vi "Lower First Letter.vi"(10 "String In":string) -> (2 "String Out":string)   [LabVIEW 2015, in "Case Manipulation.lvlib"]
uses:
  Case Manipulation.lvlib
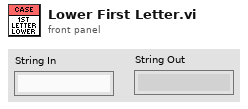
[diagram p1: front panel]
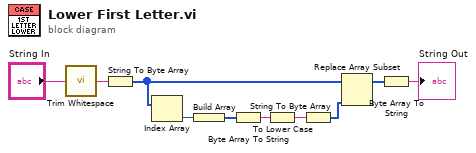
[diagram p0: block diagram]
diagram:
  n1 = call <vilib>:"Trim Whitespace.vi"("string"="String In") -> ("trimmed string"=w8:string)  [unwired: 1 in]
  n2 = String To Byte Array(string=w8) -> (unsigned byte array=w4:u8[])
  n3 = Index Array(array=w4) -> (element=w9:u8)  [unwired: 1 in]
  n4 = Build Array(w9) -> (w7:u8[])
  n5 = Byte Array To String(unsigned byte array=w7) -> (string=w6:string)
  n6 = To Lower Case(string=w6) -> (all lower case string=w5:string)
  n7 = String To Byte Array(string=w5) -> (unsigned byte array=w3:u8[])
  n8 = Replace Array Subset(array=w4, new element=w3) -> (w2:u8[])  [unwired: 1 in]
  n9 = Byte Array To String(unsigned byte array=w2) -> (string=→"String Out":string)
